vi "Module Init.vi"(8 "error in (no error)":errorcluster, 11 "Debug GUI Module in":refnum<class "Debug GUI Module.lvclass">) -> (0 "error out":errorcluster, 3 "Debug GUI Module out":refnum<class "Debug GUI Module.lvclass">)   [LabVIEW 2020, in "VolatusGUI.lvlib" / "Debug GUI Module.lvclass"]
uses:
  Debug GUI Module.lvclass
  Debug GUI Module.lvclass/Debug GUI Module.ctl
  Volatus/Module/Module.lvclass
  C:/dev/lv20CE/relink/lv-volatus/Volatus/Module/Module.lvclass
  C:/dev/lv20CE/relink/lv-volatus/VolatusGUI/Debug GUI Module/Debug GUI Module.lvclass
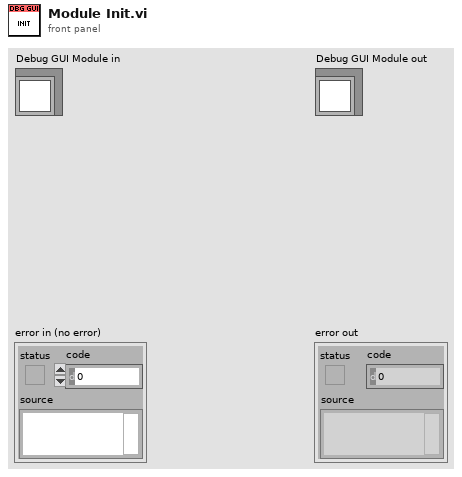
[diagram p1: front panel]
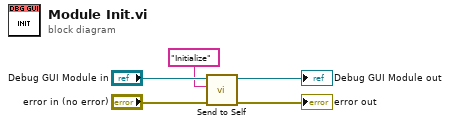
[diagram p0: block diagram]
diagram:
  n1 = call "Send to Self.vi"("error in (no error)"="error in (no error)", "Message ID"="Initialize", "Module in"="Debug GUI Module in") -> ("error out"=→"error out":errorcluster, "Module out"=→"Debug GUI Module out":refnum<class "Debug GUI Module.lvclass">)  [unwired: 7 in]
